vi "set_authorization.vi"(8 "error in (no error)":errorcluster, 10 "expire":timestamp, 11 "authorization":string) -> (0 "error out":errorcluster)   [LabVIEW 2015, in "lv-dropbox.lvlib"]
uses:
  lv-dropbox.lvlib
  private/_controls/authorization.ctl
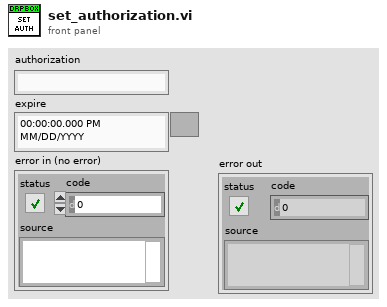
[diagram p1: front panel]
types:
  T1 = typedef "lv-dropbox.lvlib/authorization.ctl" = cluster{"authorization":string, "expire":timestamp}
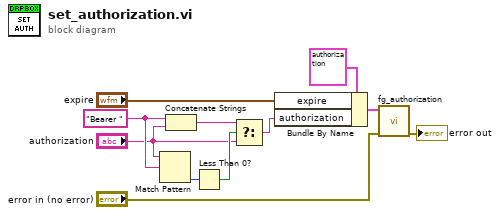
[diagram p0: block diagram]
diagram:
  w3 = "Bearer " ("string")
  n1 = Match Pattern(string="authorization", regular expression=w3) -> (offset past match=w6:i32)  [unwired: 1 in, 3 out]
  n2 = Concatenate Strings(w3, "authorization") -> (w1:string)
  n3 = Less Than 0?(x=w6) -> (x < 0?=w5:bool)
  n4 = Select(t=w1, s=w5, f="authorization") -> (s? t:f=w4:string)
  n5 = Bundle By Name(cluster=T1 {"authorization"="", "expire"=timestamp(0 s since 1904-01-01)} ("authorization in"), "expire"="expire", "authorization"=w4) -> (w8:T1)
  n6 = call "fg_authorization.vi"("error in (no error)"="error in (no error)", "authorization in"=w8) -> ("error out"=→"error out":errorcluster)  [unwired: 8 in, 1 out]
